vi "Subvi multiplexer.vi"(4 "number 8":u8, 5 "number 1":u8, 6 "number 7":u8, 7 "number 2":u8, 8 "number 6":u8, 9 "number 5":u8, 10 "number 4":u8, 11 "number 3":u8) -> (2 "result":u32)   [LabVIEW 2017]
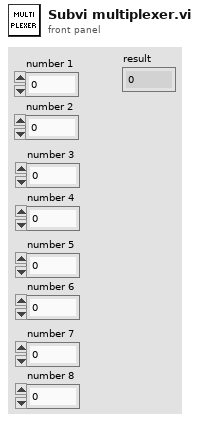
[diagram p1: front panel]
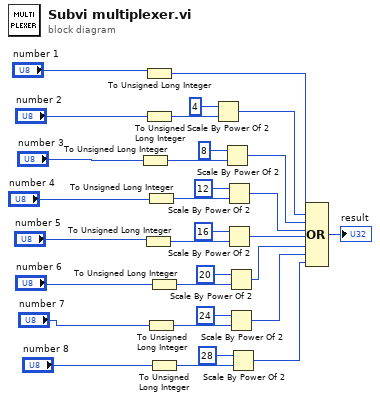
[diagram p0: block diagram]
diagram:
  n1 = To Unsigned Long Integer(number="number 3") -> (unsigned 32bit integer=w15:u32)
  n2 = To Unsigned Long Integer(number="number 5") -> (unsigned 32bit integer=w13:u32)
  n3 = To Unsigned Long Integer(number="number 1") -> (unsigned 32bit integer=w17:u32)
  n4 = To Unsigned Long Integer(number="number 2") -> (unsigned 32bit integer=w16:u32)
  n5 = To Unsigned Long Integer(number="number 4") -> (unsigned 32bit integer=w14:u32)
  n6 = To Unsigned Long Integer(number="number 7") -> (unsigned 32bit integer=w11:u32)
  n7 = To Unsigned Long Integer(number="number 6") -> (unsigned 32bit integer=w12:u32)
  n8 = To Unsigned Long Integer(number="number 8") -> (unsigned 32bit integer=w10:u32)
  n9 = Scale By Power Of 2(n=i16 4, x=w16) -> (x*2^n=w28:u32)
  n10 = Scale By Power Of 2(n=i16 8, x=w15) -> (x*2^n=w27:u32)
  n11 = Scale By Power Of 2(n=i16 12, x=w14) -> (x*2^n=w26:u32)
  n12 = Scale By Power Of 2(n=i16 16, x=w13) -> (x*2^n=w21:u32)
  n13 = Scale By Power Of 2(n=i16 20, x=w12) -> (x*2^n=w20:u32)
  n14 = Scale By Power Of 2(n=i16 24, x=w11) -> (x*2^n=w19:u32)
  n15 = Scale By Power Of 2(n=i16 28, x=w10) -> (x*2^n=w18:u32)
  n16 = Compound Arithmetic op=OR(w17, w28, w27, w26, w21, w20, w19, w18) -> (→"result":u32)
